vi "InitializeconnectGetVarOutputs.vi"(0 "Value Term Refnum":refnum<vi>, 1 "Terms[]":refnum<vi>[](array[refnum]), 5 "Error Term Refnum":refnum<vi>, 7 "InitData Term Refnum":refnum<vi>, 9 "Found Term Refnum":refnum<vi>, 11 "error in (no error)":errorcluster) -> (6 "dup Terms[]":refnum<vi>[](array[refnum]), 15 "error out":errorcluster)   [LabVIEW 2009, in "HGF_VisitorGenerator.lvlib"]
doc: "connect get variant attribute outputs.\nDoesn't connect if target terminal is not a refnum"
uses:
  HGF_VisitorGenerator.lvlib
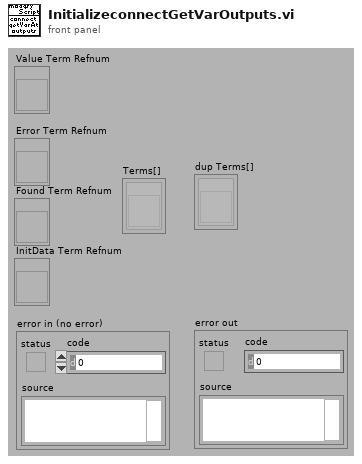
[diagram p1: front panel]
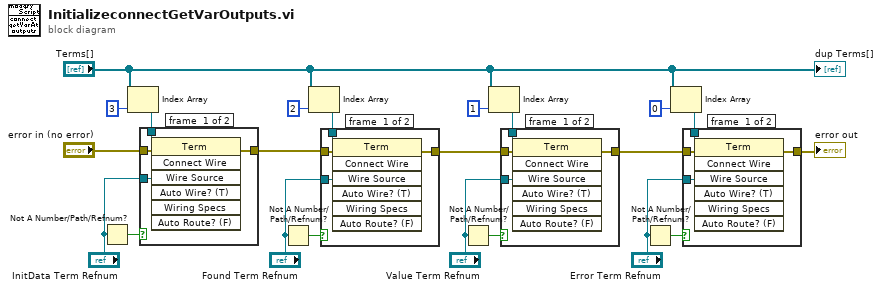
[diagram p0: block diagram]
diagram:
  n1 = Not A Number/Path/Refnum?(number/path/refnum="InitData Term Refnum") -> (NaN/Path/Refnum?=w19:bool)
  n2 = Index Array(array="Terms[]", index=3) -> (element=w22:refnum<vi>)
  n3 = case shown="False" w19 {
    tunnel: w22 -> [w26 _]
    tunnel: [w25 w27] -> w10
    tunnel: "error in (no error)" -> [w24 w27]
    tunnel: "InitData Term Refnum" -> [w23 _]
    frame #0 {
      n4 = invoke class="Term" method="Connect Wire"(reference=w26, error in=w24, "Wire Source"=w23) -> (error out=w25:errorcluster)  [unwired: 4 in, 6 out]
    }
    frame #1 {
    }
  }
  n5 = Not A Number/Path/Refnum?(number/path/refnum="Found Term Refnum") -> (NaN/Path/Refnum?=w18:bool)
  n6 = Index Array(array="Terms[]", index=2) -> (element=w14:refnum<vi>)
  n7 = case shown="False" w18 {
    tunnel: w14 -> [w31 _]
    tunnel: [w30 w32] -> w9
    tunnel: w10 -> [w29 w32]
    tunnel: "Found Term Refnum" -> [w28 _]
    frame #0 {
      n8 = invoke class="Term" method="Connect Wire"(reference=w31, error in=w29, "Wire Source"=w28) -> (error out=w30:errorcluster)  [unwired: 4 in, 6 out]
    }
    frame #1 {
    }
  }
  n9 = Not A Number/Path/Refnum?(number/path/refnum="Value Term Refnum") -> (NaN/Path/Refnum?=w17:bool)
  n10 = Index Array(array="Terms[]", index=1) -> (element=w13:refnum<vi>)
  n11 = case shown="False" w17 {
    tunnel: w13 -> [w36 _]
    tunnel: [w35 w37] -> w8
    tunnel: w9 -> [w34 w37]
    tunnel: "Value Term Refnum" -> [w33 _]
    frame #0 {
      n12 = invoke class="Term" method="Connect Wire"(reference=w36, error in=w34, "Wire Source"=w33) -> (error out=w35:errorcluster)  [unwired: 4 in, 6 out]
    }
    frame #1 {
    }
  }
  n13 = Not A Number/Path/Refnum?(number/path/refnum="Error Term Refnum") -> (NaN/Path/Refnum?=w16:bool)
  n14 = Index Array(array="Terms[]", index=0) -> (element=w11:refnum<vi>)
  n15 = case shown="False" w16 {
    tunnel: w11 -> [w41 _]
    tunnel: [w40 w42] -> w15
    tunnel: w8 -> [w39 w42]
    tunnel: "Error Term Refnum" -> [w38 _]
    frame #0 {
      n16 = invoke class="Term" method="Connect Wire"(reference=w41, error in=w39, "Wire Source"=w38) -> (error out=w40:errorcluster)  [unwired: 4 in, 6 out]
    }
    frame #1 {
    }
  }
  "error out" <- w15
  "dup Terms[]" <- "Terms[]"
